vi "DatatoGraph.vi"(0 "PluginType":string, 1 "WaveformChart in":refnum<vi>, 5 "Data":variant, 7 "PlotYScale":u32[](array[numeric]), 11 "error in (no error)":errorcluster) -> (3 "Incorrect DataType?":bool, 4 "ChromaAC Array":waveform(dbl)[](array[waveform]), 6 "ChromaDC":waveform(dbl)[](array[waveform]), 8 "NHRDC":waveform(sgl)[](array[waveform]), 10 "Array":waveform(dbl)[](array[waveform]), 14 "OutputString":string, 15 "error out":errorcluster)   [LabVIEW 2018, in "AcPwrModule.lvlib"]
doc: "This VI takes the measurement data sent via the plugins, parses it looking for data corresponding to a particular instrument and displays that data."
uses:
  AcPwrModule.lvlib
  AcPwrPlugins/ChromaAcLoad/TypeDefs/Measurements.ctl
  AcPwrPlugins/ChromaAcLoad/TypeDefs/MeasurementType.ctl
  AcPwrPlugins/NHRDCPower/TypeDefs/Measurements.ctl
  AcPwrPlugins/PacificPowerSource/TypeDefs/Measurements.ctl
  AcPwrPlugins/ChromaAcLoad/ChromaAcLoad.lvclass
  AcPwrPlugins/NHRDCPower/NHRDCPower.lvclass
  AcPwrPlugins/PacificPowerSource/PacificPowerSource.lvclass
panel:
  in  "Tab Control":enum32{"CHROMAAC", "CHROMADC", "NHRDC", "PPS"}(tab)
  out "Measurement":i32(ring)=1 items=["Voltage"=1, "Positive Peak Voltage"=2, "Positive Peak Voltage Last Fetch"=4, "Negative Peak Voltage"=8, "Negative Peak Voltage Last Fetch"=16, "Current"=32, "Positive Peak Current"=64, "Positive Peak Current Last Fetch"=128, "Negative Peak Current"=256, "Negative Peak Current Last Fetch"=512, "Power"=1024, "Positive Peak Power"=2048, "Positive Peak Power Last Fetch"=4096, "Negative Peak Power"=8192, "Negative Peak Power Last Fetch"=16384, "Timestamp"=32768, "Charge Time"=65536, "Discharge Time"=131072, "Amp Hour"=262144, "Amp Hour Time"=524288, "Amp Hour Charge"=1048576, "Amp Hour Discharge"=2097152, "Kilo Watt Hour"=4194304, "Kilo Watt Hour Time"=8388608, "Kilo Watt Hour Charge"=16777216, "Kilo Watt Hour Discharge"=33554432, "UUT Temperature"=67108864]
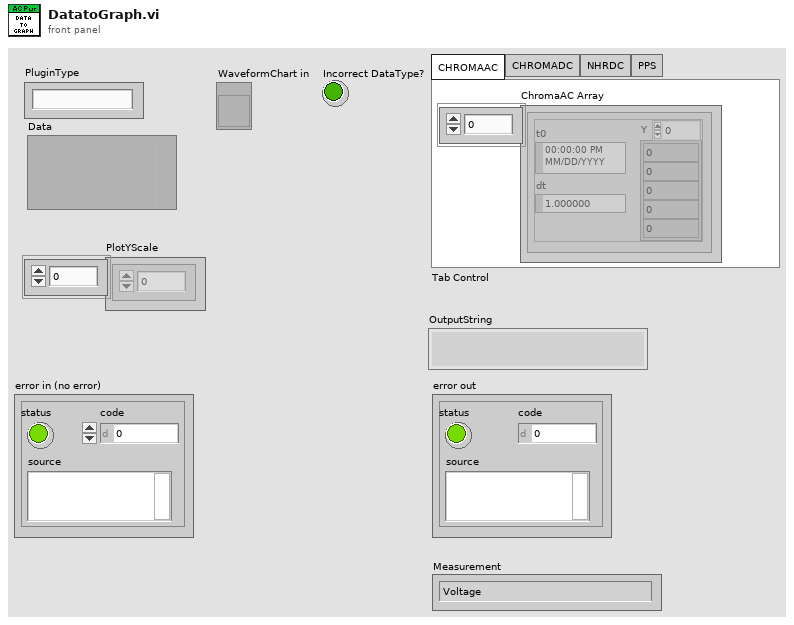
[diagram p1: front panel]
types:
  T1 = typedef "AcPwrPlugins.lvlib/PacificPowerSource.lvclass/Measurements.ctl" = cluster{"Handle":string, "Name":string, "Enabled ":bool, "Measurement Value":dbl, "Channel Name":enum16{"A", "B", "C"}, "Measurement Type ":enum16{"Voltage RMS L-N", "Voltage RMS L-L", "Frequency", "Current RMS", "Current Peak", "Crest Factor", "Power Factor", "Power VA", "Real Power"}}[]
  T2 = typedef "AcPwrPlugins.lvlib/NHRDCPower.lvclass/Measurements.ctl" = cluster{"Handle":string, "Name":string, "Enabled":bool, "Measurement Value":sgl, "btnMeasFetch":bool, "Measurement Type":i32, "Fetch Method":i32, "Fetch Time (s)":sgl}[]
  T3 = typedef "AcPwrPlugins.lvlib/ChromaAcLoad.lvclass/Measurements.ctl" = cluster{"Handle":string, "Name":string, "Enabled":bool, "Measurement Value":dbl, "Hold Peak Current Measurement":bool, "btnMeasFetch":bool, "ProtectionStatusString":string, "Measurement Type":T4}[]
  T4 = typedef "AcPwrPlugins.lvlib/ChromaAcLoad.lvclass/MeasurementType.ctl" = enum16{"Voltage (Vrms or V)", "Current (Arms or A)", "Power (W)", "Peak Voltage (V)", "Peak Current (A)", "Peak Power (W)", "Frequency (Hz)", "Resistance (Ohms)", "Voltage Overshoot (V)", "Positive Peak Current (A)", "Voltage Undershoot (V)", "Negative Peak Current (A)", "Apparent Power (VA)", "Reacitive Power (VAR)", "Voltage THD", "Power Factor", "Current's Crest Factor"}
  T5 = enum16{"Voltage RMS L-N", "Voltage RMS L-L", "Frequency", "Current RMS", "Current Peak", "Crest Factor", "Power Factor", "Power VA", "Real Power"}
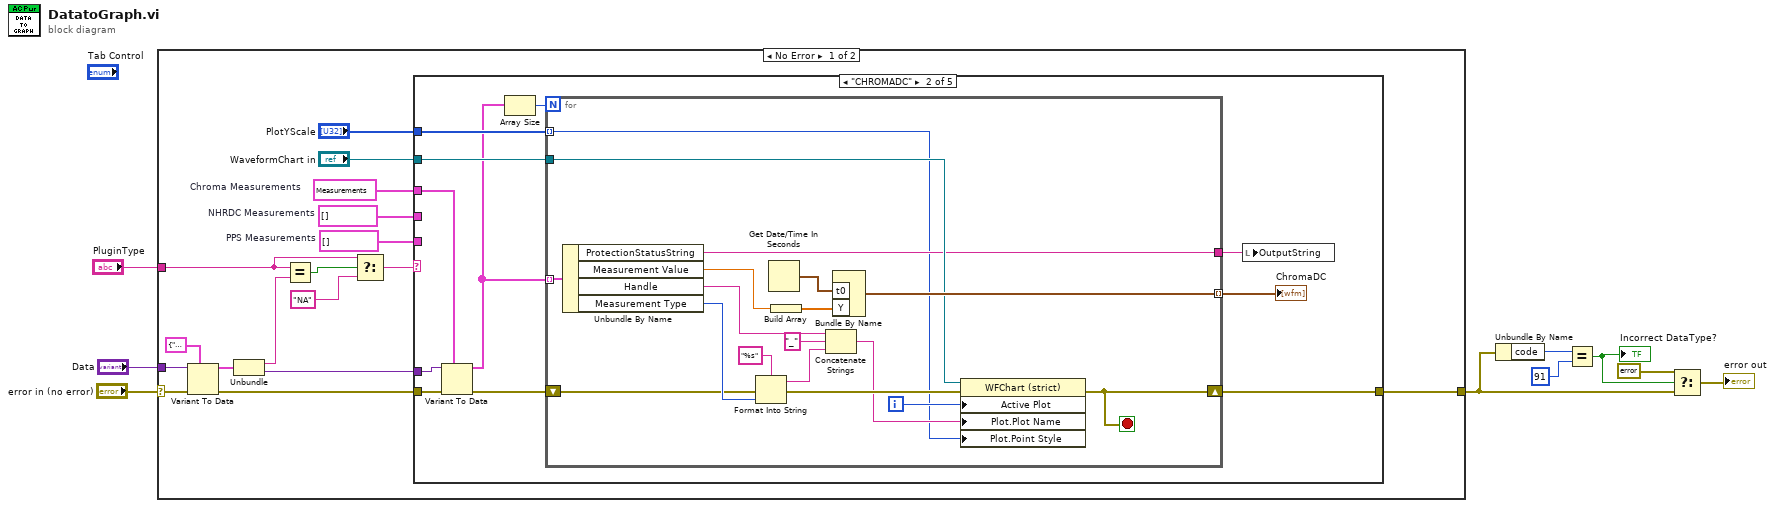
[diagram p0: block diagram]
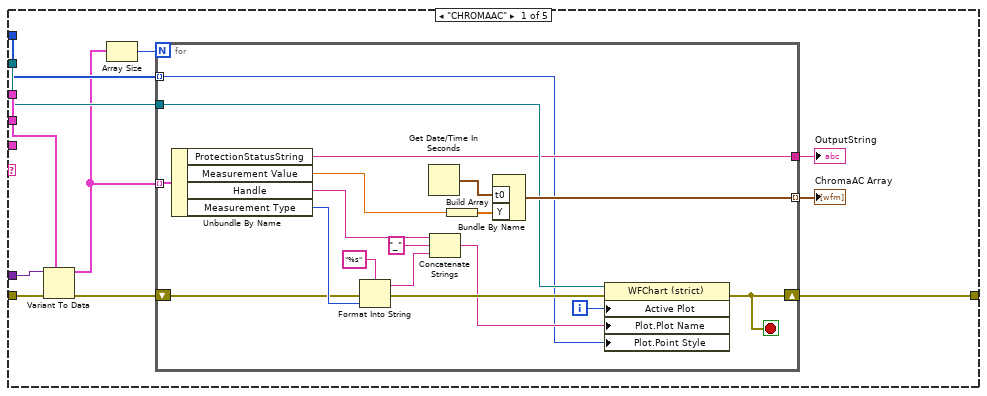
[diagram p2: hidden frame]
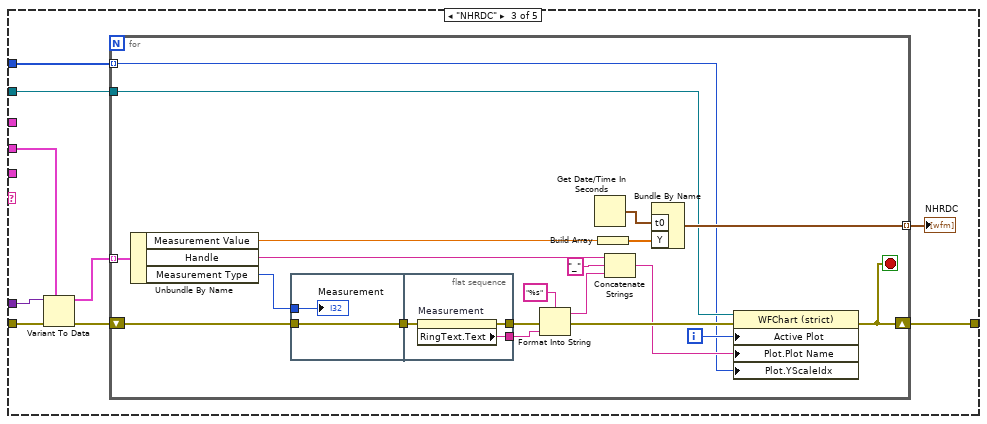
[diagram p3: hidden frame]
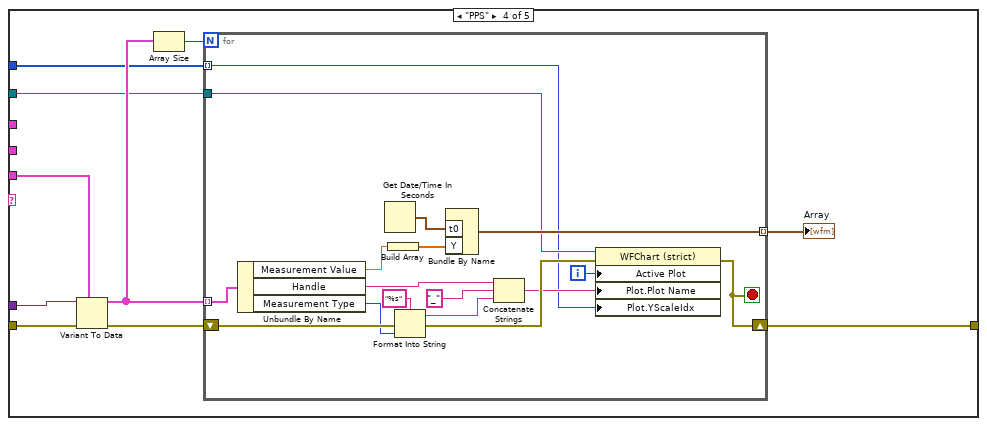
[diagram p4: hidden frame]
diagram:
  n1 = case shown="No Error" "error in (no error)" {
    selector: "error in (no error)" -> [w21 w147]
    tunnel: "Data" -> [w22 _]
    tunnel: [w25 w147] -> w2
    tunnel: "PluginType" -> [w17 _]
    frame No Error {
      w10 = T1 []  # PPS Measurements
      w13 = T2 []  # NHRDC Measurements
      w26 = T3 [{"Handle"="", "Name"="", "Enabled"=FALSE, "Measurement Value"=0.0, "Hold Peak Current Measurement"=FALSE, "btnMeasFetch"=TRUE, "ProtectionStatusString"="", "Measurement Type"=enum."Voltage (Vrms or V)"}]  # Chroma Measurements
      n2 = Variant To Data(error in=w21, type=cluster{string, "Data":variant} {"", "Data"=variant}, Variant=w22) -> (data=w23:cluster{string, "Data":variant}, error out=w20:errorcluster)
      n3 = Unbundle(w23) -> (w18:string, "Data"=w19:variant)
      n4 = Equal?(x=w17, y=w18) -> (x = y?=w16:bool)
      n5 = Select(t=w17, s=w16, f="NA") -> (s? t:f=w14:string)
      n6 = case shown="\"CHROMADC\"" w14 {
        tunnel: w26 -> [w37 w66 _ _ _]
        tunnel: w19 -> [w36 w65 w93 w128 _]
        tunnel: [w34 w63 w86 w120 w146] -> w25
        tunnel: w20 -> [w35 w64 w92 w127 w146]
        tunnel: w13 -> [_ _ w91 _ _]
        tunnel: "WaveformChart in" -> [w31 w61 w90 w122 _]
        tunnel: "PlotYScale" -> [w29 w59 w87 w121 _]
        tunnel: w10 -> [_ _ _ w123 _]
        frame "CHROMAAC" {
          n7 = Variant To Data(error in=w35, type=w37, Variant=w36) -> (data=w27:T3, error out=w33:errorcluster)
          n8 = Array Size(array=w27) -> (size(s)=w28:i32)
          n9 = for {
            N: w28 -> [_]
            shift-right: [w39] -> w34
            shift-left: w33 -> [w46]
            tunnel: w27 -> [w55] mode=indexing
            tunnel: [w54] -> w30 mode=indexing
            tunnel: w31 -> [w41]
            tunnel: [w40] -> w32
            tunnel: w29 -> [w38] mode=indexing
            i -> [w53]
            stop <- w39 stop-if-true
            n10 = Unbundle By Name(w55) -> ("ProtectionStatusString"=w40:string, "Measurement Value"=w51:dbl, "Handle"=w49:string, "Measurement Type"=w47:T4)
            n11 = Format Into String(format string="%s", error in=w46, w47) -> (resulting string=w44:string, error out=w45:errorcluster)  [unwired: 1 in]
            n12 = Get Date/Time In Seconds() -> (seconds since 1Jan1904=w52:timestamp)
            n13 = Concatenate Strings(w49, "_" ("string"), w44) -> (w43:string)
            n14 = Build Array(w51) -> (w50:dbl[])
            n15 = Bundle By Name("t0"=w52, "Y"=w50) -> (w54:waveform(dbl))  [unwired: 1 in]
            n16 = property on="Property Node" class="WFChart (strict)"(reference=w41, error in=w45, "Active Plot"=w53, "Plot.Plot Name"=w43, "Plot.Point Style"=w38) -> (error out=w39:errorcluster)  [unwired: 1 out]
          }
          "OutputString" <- w32
          "ChromaAC Array" <- w30
        }
        frame "CHROMADC" {
          n17 = Variant To Data(error in=w64, type=w66, Variant=w65) -> (data=w58:T3, error out=w62:errorcluster)
          n18 = Array Size(array=w58) -> (size(s)=w57:i32)
          n19 = for {
            N: w57 -> [_]
            shift-right: [w68] -> w63
            shift-left: w62 -> [w75]
            tunnel: w58 -> [w84] mode=indexing
            tunnel: [w83] -> w60 mode=indexing
            tunnel: w61 -> [w70]
            tunnel: [w69] -> w56
            tunnel: w59 -> [w67] mode=indexing
            i -> [w82]
            stop <- w68 stop-if-true
            n20 = Unbundle By Name(w84) -> ("ProtectionStatusString"=w69:string, "Measurement Value"=w80:dbl, "Handle"=w78:string, "Measurement Type"=w76:T4)
            n21 = Format Into String(format string="%s", error in=w75, w76) -> (resulting string=w73:string, error out=w74:errorcluster)  [unwired: 1 in]
            n22 = Get Date/Time In Seconds() -> (seconds since 1Jan1904=w81:timestamp)
            n23 = Build Array(w80) -> (w79:dbl[])
            n24 = Concatenate Strings(w78, "_" ("string"), w73) -> (w72:string)
            n25 = Bundle By Name("t0"=w81, "Y"=w79) -> (w83:waveform(dbl))  [unwired: 1 in]
            n26 = property on="Property Node" class="WFChart (strict)"(reference=w70, error in=w74, "Active Plot"=w82, "Plot.Plot Name"=w72, "Plot.Point Style"=w67) -> (error out=w68:errorcluster)  [unwired: 1 out]
          }
          "ChromaDC" <- w60
          n27 = local write "OutputString"(w56) -> ()
        }
        frame "NHRDC" {
          n28 = Variant To Data(error in=w92, type=w91, Variant=w93) -> (data=w88:T2, error out=w89:errorcluster)
          n29 = for {
            shift-right: [w96] -> w86
            shift-left: w89 -> [w100]
            tunnel: w88 -> [w113] mode=indexing
            tunnel: [w112] -> w85 mode=indexing
            tunnel: w90 -> [w97]
            tunnel: w87 -> [w94] mode=indexing
            i -> [w111]
            stop <- w96 stop-if-true
            n30 = Unbundle By Name(w113) -> ("Measurement Value"=w109:sgl, "Handle"=w107:string, "Measurement Type"=w95:i32)
            n31 = flat-sequence {
              tunnel: w100 -> [w115]
              tunnel: [w115] -> w98
              tunnel: w95 -> [w114]
              tunnel: [w118] -> w101
              tunnel: [w116] -> w99
              tunnel: w98 -> [w117]
              frame #0 {
                "Measurement" <- w114
              }
              frame #1 {
                n32 = property on="Measurement" class="Ring (strict)"(error in=w117) -> (error out=w116:errorcluster, "RingText.Text"=w118:string)  [unwired: 1 in, 1 out]
              }
            }
            n33 = Format Into String(format string="%s", error in=w99, w101) -> (resulting string=w104:string, error out=w105:errorcluster)  [unwired: 1 in]
            n34 = Get Date/Time In Seconds() -> (seconds since 1Jan1904=w110:timestamp)
            n35 = Build Array(w109) -> (w108:sgl[])
            n36 = Concatenate Strings(w107, "_" ("string"), w104) -> (w103:string)
            n37 = Bundle By Name("t0"=w110, "Y"=w108) -> (w112:waveform(sgl))  [unwired: 1 in]
            n38 = property on="Property Node" class="WFChart (strict)"(reference=w97, error in=w105, "Active Plot"=w111, "Plot.Plot Name"=w103, "Plot.YScaleIdx"=w94) -> (error out=w96:errorcluster)  [unwired: 1 out]
          }
          "NHRDC" <- w85
        }
        frame "PPS" {
          n39 = Variant To Data(error in=w127, type=w123, Variant=w128) -> (data=w124:T1, error out=w126:errorcluster)
          n40 = Array Size(array=w124) -> (size(s)=w125:i32)
          n41 = for {
            N: w125 -> [_]
            shift-right: [w132] -> w120
            shift-left: w126 -> [w133]
            tunnel: w124 -> [w145] mode=indexing
            tunnel: [w144] -> w119 mode=indexing
            tunnel: w122 -> [w130]
            tunnel: w121 -> [w129] mode=indexing
            i -> [w143]
            stop <- w132 stop-if-true
            n42 = Unbundle By Name(w145) -> ("Measurement Value"=w141:dbl, "Handle"=w139:string, "Measurement Type"=w131:T5)
            n43 = Get Date/Time In Seconds() -> (seconds since 1Jan1904=w142:timestamp)
            n44 = Build Array(w141) -> (w140:dbl[])
            n45 = Format Into String(format string="%s", error in=w133, w131) -> (resulting string=w136:string, error out=w137:errorcluster)  [unwired: 1 in]
            n46 = Bundle By Name("t0"=w142, "Y"=w140) -> (w144:waveform(dbl))  [unwired: 1 in]
            n47 = Concatenate Strings(w139, "_" ("string"), w136) -> (w135:string)
            n48 = property on="Property Node" class="WFChart (strict)"(reference=w130, error in=w137, "Active Plot"=w143, "Plot.Plot Name"=w135, "Plot.YScaleIdx"=w129) -> (error out=w132:errorcluster)  [unwired: 1 out]
          }
          "Array" <- w119
        }
        frame "NA", Default {
        }
      }
    }
    frame Error {
    }
  }
  n49 = Unbundle By Name(w2) -> ("code"=w7:i32)
  n50 = Equal?(x=w7, y=91) -> (x = y?=w5:bool)
  "Incorrect DataType?" <- w5
  n51 = Select(t=errorcluster {"status"=FALSE, "code"=0, "source"=""} ("error IO"), s=w5, f=w2) -> (s? t:f=→"error out":errorcluster)
